vi "Configuration.To String.vi"(8 "error in (no error)":errorcluster, 11 "Configuration in":refnum<class "Configuration.lvclass">) -> (0 "error out":errorcluster, 2 "String":string, 3 "Configuration out":refnum<class "Configuration.lvclass">)   [LabVIEW 2017, in "DSF Core.lvlib" / "Configuration Session.lvclass"]
uses:
  DSF Configuration API/Configuration Session.lvclass
  Configuration.lvclass
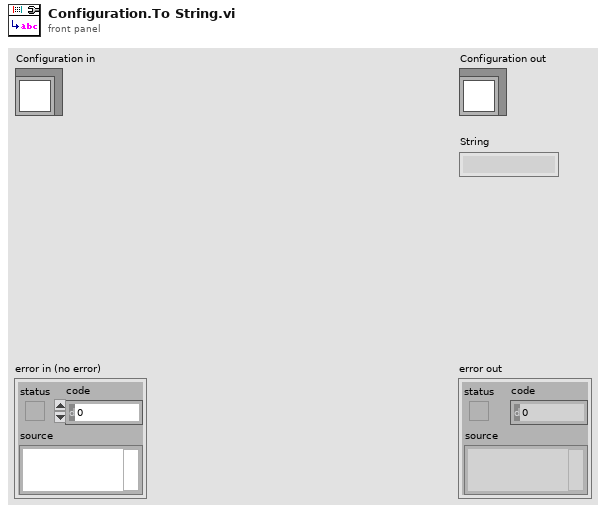
[diagram p1: front panel]
types:
  T1 = enum16{"big-endian, network order", "native, host order", "little-endian"}
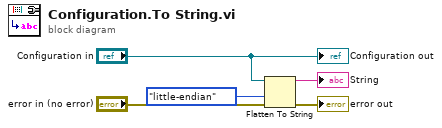
[diagram p0: block diagram]
diagram:
  n1 = Flatten To String(anything="Configuration in", byte order (0:big-endian, network order)=T1."little-endian", error in (no error)="error in (no error)") -> (data string=→"String":string, error out=→"error out":errorcluster)  [unwired: 1 in, 1 out]
  "Configuration out" <- "Configuration in"
